vi "Transmitter (My).vi"() -> ()   [LabVIEW 2015]
uses:
  <vilib>/addons/Modulation/Digital/General/MT Generate PSK System Parameters(M).vi
  <instrlib>/niUSRP/niUSRP Write Tx Data (CDB Cluster).vi
  <vilib>/addons/Modulation/niDMT.lvlib
panel:
  out "Constellation Graph":T1(graph) caption="Tx Signal Constellation"
  in  "stop":bool
  out "Symbol Rate\n[symbols/sec]":dbl=500000.0 format="%#.6p"
  in  "filter parameters":T2={"Alpha"=0.5, "Filter Length"=6, "TX Filter"=enum."Root Raised Cos"} {"Alpha" format="%.2f"}
  in  "PN Sequence Order":i32=10
  out "Frame Size [samples]":i32=4092
  in  "Choose b/w  BPSK and QPSK Format":enum32{"BPSK", "QPSK"}(tab)=enum."QPSK" caption="PSK"
  in  "BPSK System Parameters":T3={"Samples per Symbol"=8, "symbol map"=[]} {"symbol map" format="%.3f"}
  in  "QPSK System Parameters":T3={"Samples per Symbol"=8, "symbol map"=[]} {"symbol map" format="%.3f"}
  in  "device name":refnum<k15>="192.168.10.5"
  in  "IQ Sampling\nRate [S/sec]":dbl=500000.0 format="%#.6p"
  in  "Carrier\nFrequency [Hz]":dbl=915000000.0 format="%#.6p"
  in  "Gain [dB]":dbl=12.0 format="%#.6p"
  in  "Active Antenna":string(combo)="TX1"
  out "IQ Sampling\nRate [S/sec] (actual)":dbl=500000.0 format="%#.6p"
  out "Carrier Frequency \n[Hz] (actual)":dbl=915000000.0 format="%#.6p"
  out "Gain [dB] (actual)":dbl=12.0 format="%#.6p"
  in  "Enabled Channel":string(combo)="0"
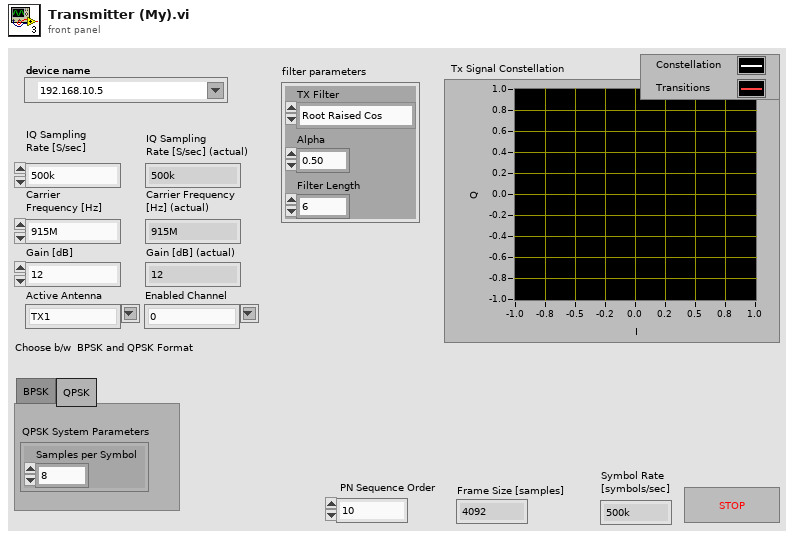
[diagram p1: front panel]
types:
  T1 = cluster{"constellation":dbl[], "oversampled data":dbl[]}[]
  T2 = cluster{"Alpha":dbl, "Filter Length":i32, "TX Filter":enum16{"none", "Raised Cosine", "Root Raised Cos", "Gaussian"}}
  T3 = cluster{"Samples per Symbol":i32, "symbol map":cdb[]}
  T4 = cluster{"samples per symbol (16)":i32, "symbol map":cdb[], "differential PSK":enum16{"disable", "enable"}, "PSK type":u16}
  T5 = typedef "niAMT.lvlib/Complex Data Waveform.ctl" = cluster{"t0":dbl, "dt":dbl, "Y":cdb[]}
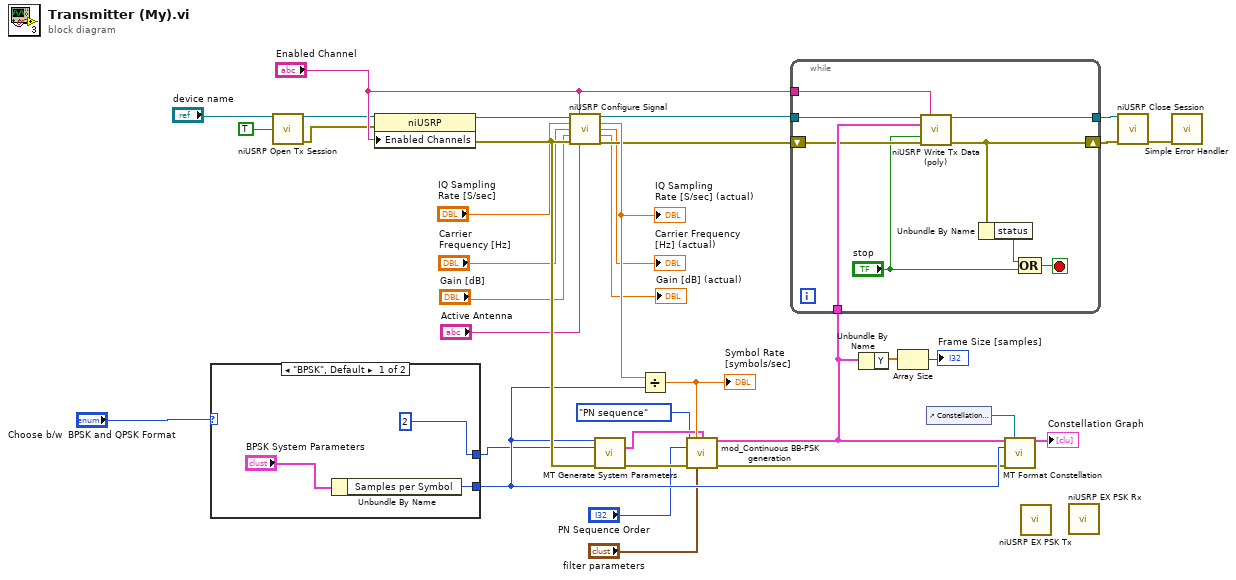
[diagram p0: block diagram]
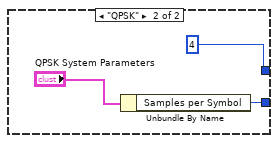
[diagram p2: hidden frame]
diagram:
  n1 = case shown="\"BPSK\", Default" "Choose b/w  BPSK and QPSK Format" {
    tunnel: [w37 w40] -> w29
    tunnel: [2 4] -> w1
    frame "BPSK", Default {
      n2 = Unbundle By Name("BPSK System Parameters") -> ("Samples per Symbol"=w37:i32)
    }
    frame "QPSK" {
      n3 = Unbundle By Name("QPSK System Parameters") -> ("Samples per Symbol"=w40:i32)
    }
  }
  n4 = call <instrlib>:"niUSRP Open Tx Session.vi"("device names"="device name", "reset"=TRUE) -> ("session handle out"=w30:refnum<k15>, "error out"=w31:errorcluster)  [unwired: 12 in]
  n5 = property class="niUSRP"(reference=w30, error in=w31, "Enabled Channels"="Enabled Channel") -> (reference out=w32:refnum<k15>, error out=w33:errorcluster)
  n6 = call <instrlib>:"niUSRP Configure Signal.vi"("session handle"=w32, "channel list"="Enabled Channel", "IQ rate"="IQ Sampling\nRate [S/sec]", "carrier frequency"="Carrier\nFrequency [Hz]", "gain"="Gain [dB]", "error in (no error)"=w33, "active antenna"="Active Antenna") -> ("session handle out"=w26:refnum<k15>, "coerced IQ rate"=w28:dbl, "coerced carrier frequency"=→"Carrier Frequency \n[Hz] (actual)":dbl, "coerced gain"=→"Gain [dB] (actual)":dbl, "error out"=w27:errorcluster)  [unwired: 4 in]
  "IQ Sampling\nRate [S/sec] (actual)" <- w28
  n7 = call-poly <vilib>:"MT Generate System Parameters.vi"("samples per symbol (16)"=w29, "M-PSK (4)"=w1, "error in (no error)"=w33) -> ("PSK system parameters"=w11:T4, "error out"=w10:errorcluster)  [unwired: 10 in, 1 out]
  n8 = Divide(x=w28, y=w29) -> (x/y=w12:dbl)
  "Symbol Rate\n[symbols/sec]" <- w12
  n9 = call <vilib>:"mod_Continuous BB-PSK generation.vi"("bit stream type"=enum32{"PN sequence", "user-defined pattern"}."PN sequence", "Symbol Rate, Hz"=w12, "Custom-PSK Parameters"=w11, "PN Sequence Order"="PN Sequence Order", "error in (no error)"=w10, "filter parameters"="filter parameters") -> ("output complex waveform"=w13:T5, "error out"=w18:errorcluster)  [unwired: 7 in, 1 out]
  n10 = while {
    tunnel: [w46] -> w15
    tunnel: w26 -> [w49]
    shift-right: [w42] -> w14
    shift-left: w27 -> [w47]
    tunnel: w13 -> [w48]
    tunnel: "Enabled Channel" -> [w41]
    stop <- w45 stop-if-true
    n11 = call-poly <instrlib>:"niUSRP Write Tx Data (poly).vi"("session handle"=w49, "channel list"=w41, "data"=w48, "end of data?"="stop", "error in (no error)"=w47) -> ("session handle out"=w46:refnum<k15>, "error out"=w42:errorcluster)  [unwired: 9 in]
    n12 = Unbundle By Name(w42) -> ("status"=w44:bool)
    n13 = Compound Arithmetic op=OR(w44, "stop") -> (w45:bool)
  }
  n14 = Unbundle By Name(w13) -> ("Y"=w4:cdb[])
  n15 = Array Size(array=w4) -> (size(s)=→"Frame Size [samples]":i32)
  n16 = control-ref of="Constellation Graph"() -> (w2:refnum<vi>)
  n17 = call <vilib>:"MT Format Constellation.vi"("waveform"=w13, "constellation reference"=w2, "samples per symbol"=w29, "error in (no error)"=w18) -> ("constellation graph"=→"Constellation Graph":T1)  [unwired: 10 in, 1 out]
  n18 = call "niUSRP EX PSK Tx.vi"() -> ()  [unwired: 1 in]
  n19 = call "niUSRP EX PSK Rx.vi"() -> ()  [unwired: 1 in]
  n20 = call <instrlib>:"niUSRP Close Session.vi"("session handle"=w15, "error in (no error)"=w14) -> ("error out"=w16:errorcluster)  [unwired: 13 in]
  n21 = call <vilib>:"Simple Error Handler.vi"("error in (no error)"=w16) -> ()  [unwired: 4 in, 5 out]
